vi "ManualL1ControlNoLoop.vi"() -> ()   [LabVIEW 2012]
uses:
  <vilib>/Utility/NIReport.llb/NI_report.lvclass
  <vilib>/Utility/NIReport.llb/HTML/NI_HTML.lvclass
panel:
  in  "Adder B0":u32=255 max=255 step=1
  in  "Adder B1":u32=255 max=255 step=1
  in  "Adder C0":u32=255 max=255 step=1
  in  "Adder C1":u32=255 max=255 step=1
  in  "Adder A0":u32=27 max=255 step=1
  in  "Adder A1":u32=12 max=255 step=1
  in  "Adder B 1":u32(slide)=255 max=255 step=1 scale=0.0..255.0
  in  "Adder A 1":u32(slide)=1 max=255 step=1 scale=0.0..255.0
  in  "Adder C 1":u32(slide)=255 max=255 step=1 scale=0.0..255.0
  out "Data out 0":string
  out "IPR value 0":i32
  out "hex 7":string="3400"
  out "hex 6":string="7BF"
  out "hex 5":string="FFF7"
  out "hex 4":string="FFFF"
  out "hex 3":string="1B0C"
  out "hex 2":string="FFFF"
  out "hex":string="2AAA"
  out "Data out 1":string
  out "IPR value 1":i32
  in  "Adder B 0":u32(slide)=255 max=255 step=1 scale=0.0..255.0
  in  "Adder A 0":u32(slide)=255 max=255 step=1 scale=0.0..255.0
  in  "Adder C 0":u32(slide)=255 max=255 step=1 scale=0.0..255.0
  in  "Instrument VISA in":T1={"AWG VISA"="AgilentGenerator1", "Oscilloscope  VISA "="AgilentOsciloscope", "Integration Board IP"="172.16.17.48", "connection ID"=refnum, "report out"=refnum, "report file path"=path "C:/Documents and Settings/CTA_LAB01/Desktop/L0_Asic/L0 Asic Test Data"}
  in  "SingleIN/#Combination":bool=TRUE
  in  "Combination":i32 min=0 max=127 step=1 format="%b"
  in  "! All Channels \n(false activates all channels)":bool=TRUE
  in  "Enable  L1 single  Input":i32(slide)=4 scale=0.0..6.0
  in  "error in":errorcluster
  out "data out serial":string="writtingwritting2"
  out "error out":errorcluster
  out "REG Array":u32[](array[numeric])=[10922, 65535, 6924, 65535, 65527, 1983, 13312]
  in  "Register Adress 96":bool[](array[boolean])=[FALSE, TRUE, FALSE, TRUE, FALSE, TRUE, FALSE, TRUE, FALSE, TRUE, FALSE, TRUE, FALSE, TRUE, FALSE, FALSE]
  out "REG 96":u32=10922
  out "?":bool[](array[boolean])=[TRUE, TRUE, TRUE, TRUE, TRUE, TRUE, TRUE, TRUE, TRUE, TRUE, TRUE, TRUE, TRUE, TRUE, TRUE, TRUE, FALSE, FALSE, FALSE, FALSE, FALSE, FALSE, FALSE, FALSE, FALSE, FALSE, FALSE, FALSE, FALSE, FALSE, FALSE, FALSE, FALSE, FALSE, FALSE, FALSE, FALSE, FALSE, FALSE, FALSE, FALSE, FALSE, FALSE, FALSE, FALSE, FALSE, FALSE, FALSE, FALSE, FALSE, FALSE, FALSE, FALSE, FALSE, FALSE, FALSE, FALSE, FALSE, FALSE, FALSE, FALSE, FALSE, FALSE, FALSE]
  out "REG 99":u32=65535
  out "?":bool[](array[boolean])=[FALSE, FALSE, TRUE, TRUE, FALSE, FALSE, FALSE, FALSE, TRUE, TRUE, FALSE, TRUE, TRUE, FALSE, FALSE, FALSE, FALSE, FALSE, FALSE, FALSE, FALSE, FALSE, FALSE, FALSE, FALSE, FALSE, FALSE, FALSE, FALSE, FALSE, FALSE, FALSE, FALSE, FALSE, FALSE, FALSE, FALSE, FALSE, FALSE, FALSE, FALSE, FALSE, FALSE, FALSE, FALSE, FALSE, FALSE, FALSE, FALSE, FALSE, FALSE, FALSE, FALSE, FALSE, FALSE, FALSE, FALSE, FALSE, FALSE, FALSE, FALSE, FALSE, FALSE, FALSE]
  out "REG 98":u32=6924
  out "?":bool[](array[boolean])=[TRUE, TRUE, TRUE, TRUE, TRUE, TRUE, TRUE, TRUE, TRUE, TRUE, TRUE, TRUE, TRUE, TRUE, TRUE, TRUE, FALSE, FALSE, FALSE, FALSE, FALSE, FALSE, FALSE, FALSE, FALSE, FALSE, FALSE, FALSE, FALSE, FALSE, FALSE, FALSE, FALSE, FALSE, FALSE, FALSE, FALSE, FALSE, FALSE, FALSE, FALSE, FALSE, FALSE, FALSE, FALSE, FALSE, FALSE, FALSE, FALSE, FALSE, FALSE, FALSE, FALSE, FALSE, FALSE, FALSE, FALSE, FALSE, FALSE, FALSE, FALSE, FALSE, FALSE, FALSE]
  out "REG 97":u32=65535
  in  "Register Adress 102":bool[](array[boolean])=[FALSE, FALSE, FALSE, FALSE, FALSE, FALSE, FALSE, FALSE, FALSE, FALSE, TRUE, FALSE, TRUE, TRUE, FALSE, FALSE]
  out "REG 102":u32=13312
  in  "Register Adress 101":bool[](array[boolean])=[TRUE, TRUE, TRUE, TRUE, TRUE, TRUE, FALSE, TRUE, TRUE, TRUE, TRUE, FALSE, FALSE, FALSE, FALSE, FALSE]
  out "REG 101":u32=1983
  in  "Register Adress 100":bool[](array[boolean])=[TRUE, TRUE, TRUE, FALSE, TRUE, TRUE, TRUE, TRUE, TRUE, TRUE, TRUE, TRUE, TRUE, TRUE, TRUE, TRUE]
  out "REG 100":u32=65527
  # "0           1            2"
  # "DAC_TH0"
  # "DAC_TH1"
  # "DAC_TH2"
  # "DAC_TH3"
  # "DAC_TH4"
  # "DAC_TH5"
  # "Unused"
  # "DAC_MUX_ENA"
  # "ADDER_C"
  # "LSB"
  # "MSB"
  # "ADDER_A"
  # "LSB"
  # "MSB"
  # "ADDER_B"
  # "LSB"
  # "MSB"
  # "a             b            c"
  # "a             b            c"
  # "a             b            c"
  # "a             b            c"
  # "a             b            c"
  # "Unused"
  # "CH0"
  # "CH1"
  # "CH2"
  # "CH3"
  # "CH4"
  # "a             b            c"
  # "a             b            c"
  # "ENA_0  ENA_1"
  # "ENA_0  ENA_1"
  # "BUFF\nENA"
  # "R       E       S      E        R     V        E      D"
  # "CH5"
  # "CH6"
  # "MUX"
  # "LVDS"
  # "R               E               S               E                  R                V             E              D"
  # "0            1            2            3           4             5"
  # "DAC _IB"
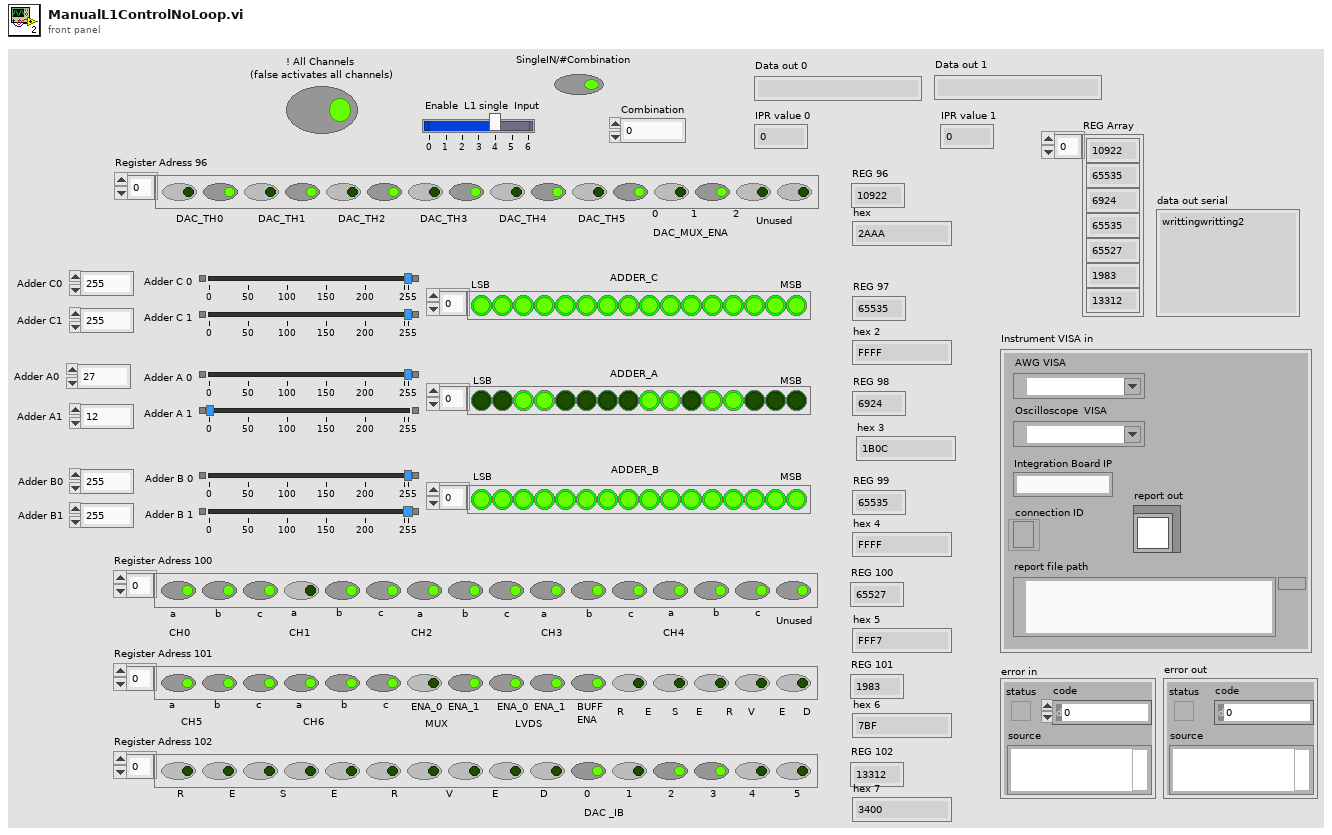
[diagram p1: front panel]
types:
  T1 = cluster{"AWG VISA":refnum<visa-resource-name>, "Oscilloscope  VISA ":refnum<visa-resource-name>, "Integration Board IP":string, "connection ID":refnum<k5>, "report out":refnum<class "NI_report.lvclass">, "report file path":path}
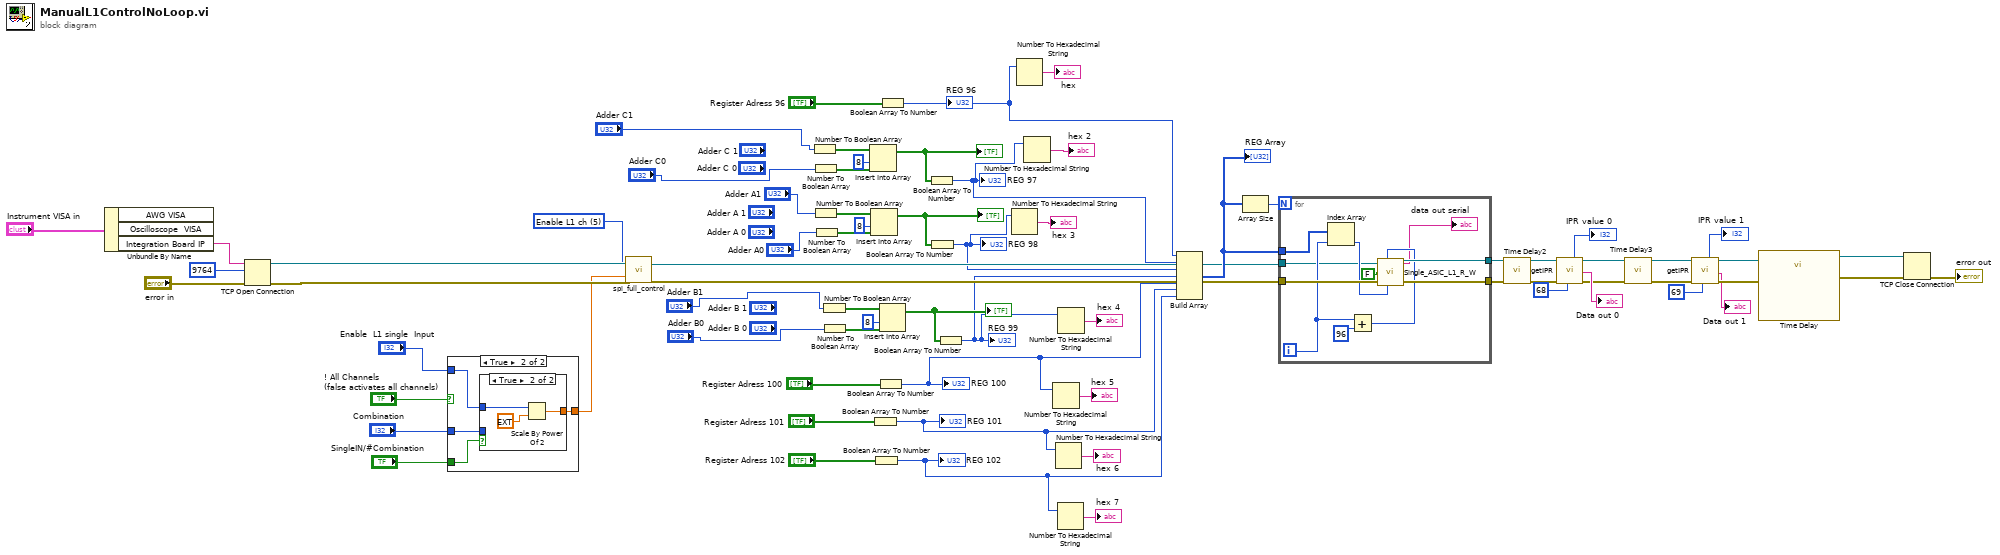
[diagram p0: block diagram]
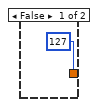
[diagram p2: hidden frame]
diagram:
  w39 = u16 5 items=["Attenuation", "Clipping", "Enable channel", "Delay line", "ASIC", "Enable L1 ch", "ASIC L1"] ("Device")
  n1 = Unbundle By Name("Instrument VISA in") -> ("Integration Board IP"=w67:string)  [unwired: 2 out]
  n2 = TCP Open Connection(address=w67, remote port or service name=9764, error in (no error)="error in") -> (connection ID=w63:refnum<k5>, error out=w62:errorcluster)  [unwired: 2 in]
  n3 = case shown="True" "! All Channels \n(false activates all channels)" {
    tunnel: [127 ("Register or channel") w72] -> w40
    tunnel: "Enable  L1 single  Input" -> [_ w73]
    tunnel: "Combination" -> [_ w71]
    tunnel: "SingleIN/#Combination" -> [_ w70]
    frame False {
    }
    frame True {
      n4 = case shown="True" w70 {
        tunnel: w73 -> [_ w76]
        tunnel: [w74 w75] -> w72
        tunnel: w71 -> [w74 _]
        frame False {
        }
        frame True {
          n5 = Scale By Power Of 2(n=w76, x=ext 1.0) -> (x*2^n=w75:ext)
        }
      }
    }
  }
  n6 = call "spi_full_control.vi"("connection ID"=w63, "Device"=w39, "Data"=w40, "error out 3"=w62) -> ("connection ID out"=w34:refnum<k5>, "error out 2"=w35:errorcluster)  [unwired: 8 in, 6 out]
  n7 = Number To Boolean Array(number="Adder C1") -> (Boolean array=w56:bool[])
  n8 = Number To Boolean Array(number="Adder C0") -> (Boolean array=w55:bool[])
  n9 = Number To Boolean Array(number="Adder A1") -> (Boolean array=w52:bool[])
  n10 = Number To Boolean Array(number="Adder A0") -> (Boolean array=w51:bool[])
  n11 = Number To Boolean Array(number="Adder B1") -> (Boolean array=w48:bool[])
  n12 = Number To Boolean Array(number="Adder B0") -> (Boolean array=w47:bool[])
  n13 = Insert Into Array(array=w56, index=8, new element=w55) -> (w54:bool[])
  "?" <- w54
  n14 = Insert Into Array(array=w52, index=8, new element=w51) -> (w50:bool[])
  "?" <- w50
  n15 = Boolean Array To Number(Boolean array="Register Adress 101") -> (number=w22:u32)
  "REG 101" <- w22
  n16 = Boolean Array To Number(Boolean array="Register Adress 102") -> (number=w20:u32)
  "REG 102" <- w20
  n17 = Boolean Array To Number(Boolean array="Register Adress 100") -> (number=w24:u32)
  "REG 100" <- w24
  n18 = Insert Into Array(array=w48, index=8, new element=w47) -> (w46:bool[])
  "?" <- w46
  n19 = Boolean Array To Number(Boolean array="Register Adress 96") -> (number=w32:u32)
  "REG 96" <- w32
  n20 = Boolean Array To Number(Boolean array=w54) -> (number=w29:u32)
  "REG 97" <- w29
  n21 = Boolean Array To Number(Boolean array=w50) -> (number=w28:u32)
  "REG 98" <- w28
  n22 = Boolean Array To Number(Boolean array=w46) -> (number=w26:u32)
  "REG 99" <- w26
  n23 = Number To Hexadecimal String(2:w28) -> (0:→"hex 3":string)  [unwired: 1 in]
  n24 = Number To Hexadecimal String(2:w32) -> (0:→"hex":string)  [unwired: 1 in]
  n25 = Number To Hexadecimal String(2:w29) -> (0:→"hex 2":string)  [unwired: 1 in]
  n26 = Number To Hexadecimal String(2:w24) -> (0:→"hex 5":string)  [unwired: 1 in]
  n27 = Number To Hexadecimal String(2:w22) -> (0:→"hex 6":string)  [unwired: 1 in]
  n28 = Number To Hexadecimal String(2:w20) -> (0:→"hex 7":string)  [unwired: 1 in]
  n29 = Number To Hexadecimal String(2:w26) -> (0:→"hex 4":string)  [unwired: 1 in]
  n30 = Build Array(w32, w29, w28, w26, w24, w22, w20) -> (w42:u32[])
  "REG Array" <- w42
  n31 = Array Size(array=w42) -> (size(s)=w43:i32)
  n32 = for {
    N: w43 -> [_]
    tunnel: w35 -> [w88]
    tunnel: w42 -> [w87]
    tunnel: [w86] -> w10
    tunnel: [w85] -> w12
    tunnel: w34 -> [w78]
    i -> [w81]
    n33 = Index Array(array=w87, index=w81) -> (element=w84:u32)
    n34 = Add(x=w81, y=96) -> (x+y=w82:i32)
    n35 = call "Single_ASIC_L1_R_W.vi"("connection ID"=w78, "Register or channel"=w82, "RD/#WR"=FALSE, "error in (no error)"=w88, "Data"=w84) -> ("data out serial"=→"data out serial":string, "connection ID out"=w86:refnum<k5>, "error out"=w85:errorcluster)  [unwired: 1 in, 1 out]
  }
  n36 = call "Time Delay2"("error in (no error)"=w12) -> ("error out"=w8:errorcluster)  [unwired: 10 in]
  n37 = call "getIPR.vi"("Address"=68, "error in"=w8, "connection ID"=w10) -> ("error out"=w11:errorcluster, "Data"=→"Data out 0":string, "connection ID out"=w9:refnum<k5>, "IPR_count"=→"IPR value 0":u32)  [unwired: 5 in]
  n38 = call "Time Delay3"("error in (no error)"=w11) -> ("error out"=w7:errorcluster)  [unwired: 10 in]
  n39 = call "getIPR.vi"("Address"=69, "error in"=w7, "connection ID"=w9) -> ("error out"=w19:errorcluster, "Data"=→"Data out 1":string, "connection ID out"=w60:refnum<k5>, "IPR_count"=→"IPR value 1":u32)  [unwired: 5 in]
  n40 = call "Time Delay"("error in (no error)"=w19) -> ("error out"=w61:errorcluster)  [unwired: 10 in]
  n41 = TCP Close Connection(connection ID=w60, error in (no error)=w61) -> (error out=→"error out":errorcluster)  [unwired: 1 in, 1 out]
